vi "ADAM_scan_table.vi"() -> ()   [LabVIEW 2022 SP3]
uses:
  <vilib>/Utility/miscctls.llb/LVRowAndColumnUnsignedTypeDef.ctl
  Anemometry/Anemometry Sub Vis/Controls/Serveds.ctl
  ADAM Client/Sub VIs/ADAM Controls/Module_type_ADAM.ctl
  ADAM Client/Sub VIs/ADAM Controls/Traverse_Level_State.ctl
  Anemometry/Anemometry Sub Vis/Controls/Post_Process.ctl
  ADAM Client/Sub VIs/ADAM Controls/Channel_State.ctl
  ADAM Client/Sub VIs/ADAM Controls/Ch_description_ADAM.ctl
  ADAM Client/Sub VIs/ADAM Controls/Function_ADAM.ctl
  ADAM Client/Sub VIs/ADAM Controls/Calib_type_ADAM.ctl
  ADAM Client/Sub VIs/ADAM Controls/Address.ctl
  700e9d19-378c-4c45-b55c-3bbad4659b44.vi
  Anemometry/Anemometry Sub Vis/Globals/Preference_global.vi
  ADAM_Global.vi
  Sub VI's/Channel_Description_Global.vi
  Anemometry/Anemometry Sub Vis/Globals/Meas_global.vi
  Sub VI's/Logged_Data_real_Global.vi
  Anemometry/Anemometry Sub Vis/Globals/Gas_management_global.vi
  Anemometry/Anemometry Sub Vis/Globals/Constants_global.vi
  <vilib>/Comparison/Less/Less Functor/Less Functor.lvclass
panel:
  in  "openSetupFolder":bool
  out "Scan:Padding:(ms)":i32
  in  "launchStatus":bool
  in  "launchTiming":bool
  out "lastScan":dbl caption="Last Scan" format="%_4fs"
  out "scanNum":i32 caption="Scan Number"
  out "enunciator":string caption="Current Process"
  in  "launchEditor":bool
  in  "flushChannelErrors":bool
  in  "stopAll":bool
  out "Talking Modules":string[][](table)
  out "Channel Errors":string[][](table)
  in  "Reconfigure Gills":bool
  in  "Log full Res Data":bool
  out "Duty No":u16 format="%016b"
  in  "Save Current setup":bool=TRUE
  in  "Load setup from file":bool
  out "ADAM scan comments":string
  out "History length":i32=250
  in  "stop":bool
  out "Results":dbl[](array[numeric]) format="%.3f"
  out "Titles":string[](array[string])
  # "The default value for this\nis saved in Scan_mode.txt"
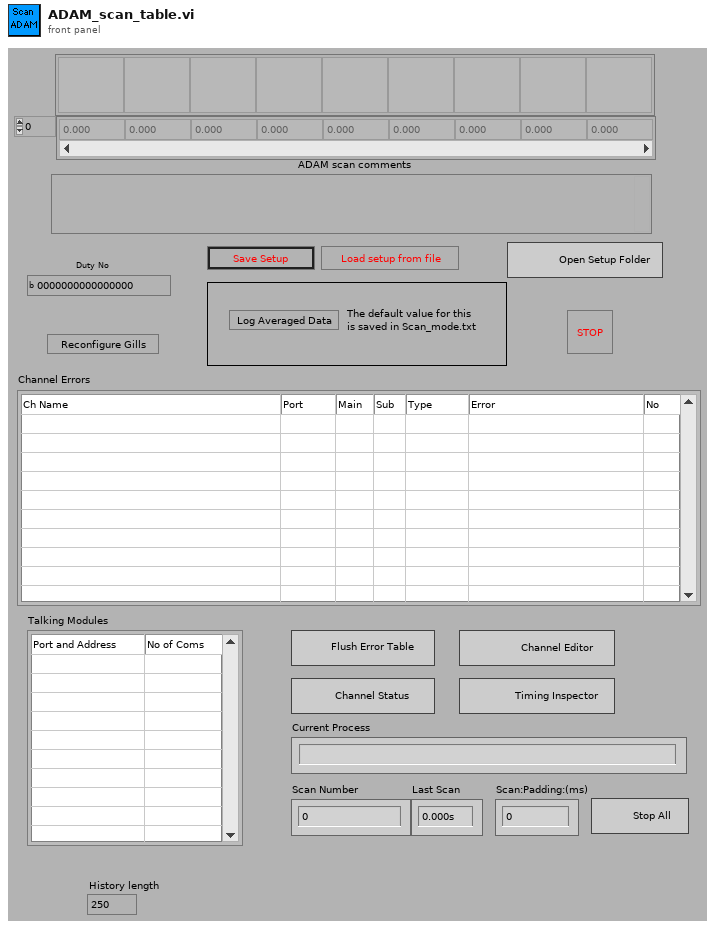
[diagram p1: front panel]
types:
  T1 = typedef "LVRowAndColumnUnsignedTypeDef.ctl" = cluster{"Row":u32, "Column":u32}
  T2 = enum16{"Load ADAM setup from excel file", "Save ADAM setup to excel file"}
  T3 = typedef "Serveds.ctl" = enum16{"Read Global", "Load Global From File"}
  T4 = typedef "Module_type_ADAM.ctl" = string
  T5 = typedef "Traverse_Level_State.ctl" = enum16{"Running", "Complete"}
  T6 = typedef "Post_Process.ctl" = enum16{"Take New Data", "Post Process Raw Data File"}
  T7 = typedef "Channel_State.ctl" = enum16{"On", "Off", "Always On", "Always Off"}
  T8 = enum32{"Invalid", "Standard", "Closed", "Hidden", "Minimized", "Maximized"}
  T9 = enum16{"Append to Global", "Read Global then Clear"}
  T10 = typedef "Ch_description_ADAM.ctl" = cluster{"Ch Name":string, "Type":T4, "Function":T11, "Ch State":T7, "Calibration type":T12, "A":dbl, "B":dbl, "C":dbl, "D":dbl, "Comments":string, "Address":T13, "String":string, "Duty":u16}
  T11 = typedef "Function_ADAM.ctl" = enum16{"Analogue Input", "Digital Input", "Event counter", "Event rate", "Analogue Output", "Digital Output", "Relay Output"}
  T12 = typedef "Calib_type_ADAM.ctl" = string
  T13 = typedef "Address.ctl" = cluster{"Main":i32, "Ch.":i32, "Sub":i32, "Port Name":string}
  T14 = enum16{"On", "Off", "Always On", "Always Off", "Delete"}
  T15 = typedef "Client_State_Cluster.ctl" = cluster{"Client Name":string, "Traverse level State":T5, "People to Email":string[], "Next Contact Time":dbl}
  T16 = typedef "LVDateTimeRec.ctl" = cluster{"fractional second":dbl, "second":i32, "minute":i32, "hour":i32, "day of month":i32, "month":i32, "year":i32, "day of week":i32, "day of year":i32, "DST":i32}
  T17 = typedef "ADAM_Comparitor.ctl" = cluster{"Ch to Monitor":string, "Channels to Kill":string, "Warn if Above":dbl, "Warn if Below":dbl, "Kill if Above":dbl, "Kill if Below":dbl, "Hysteresis Margin":dbl, "Averaging TIme (s)":dbl, "Warn Status":bool, "Kill Status":bool, "Extra Email addresses":string}
  T18 = cluster{"Channel Names":string[], "Last Updated":dbl[]}
  T19 = typedef "Update_scan_value.ctl" = cluster{"Channel Name":string, "New Value":dbl, "!Auto_Off":bool}
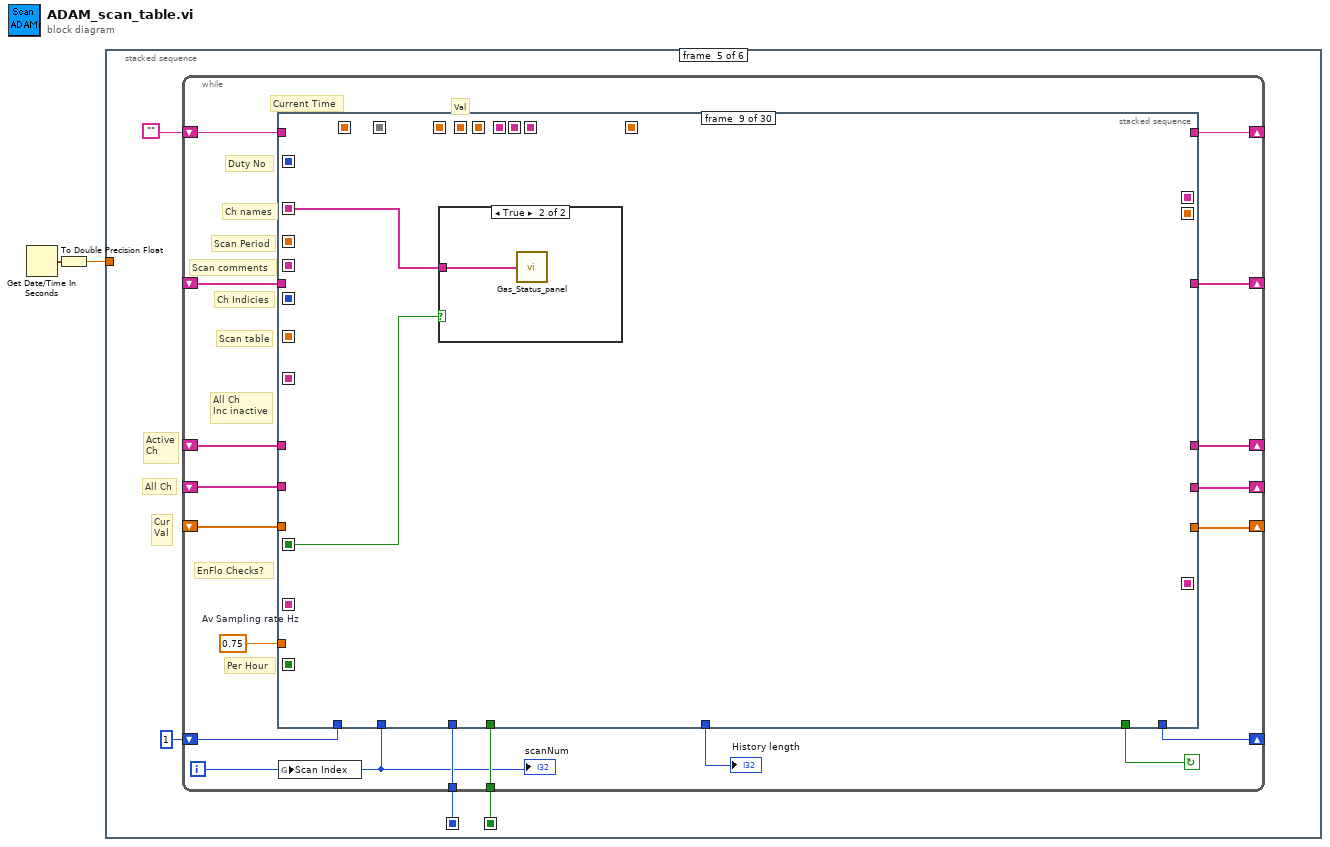
[diagram p0: block diagram]
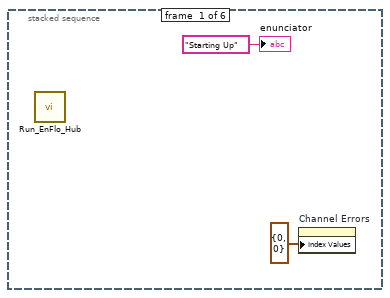
[diagram p2: hidden frame]
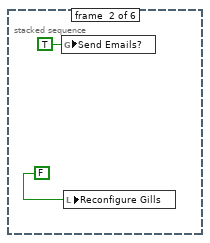
[diagram p3: hidden frame]
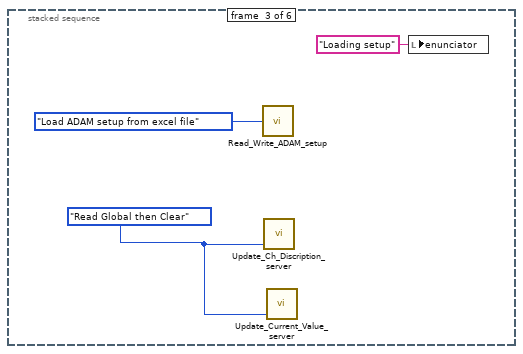
[diagram p4: hidden frame]
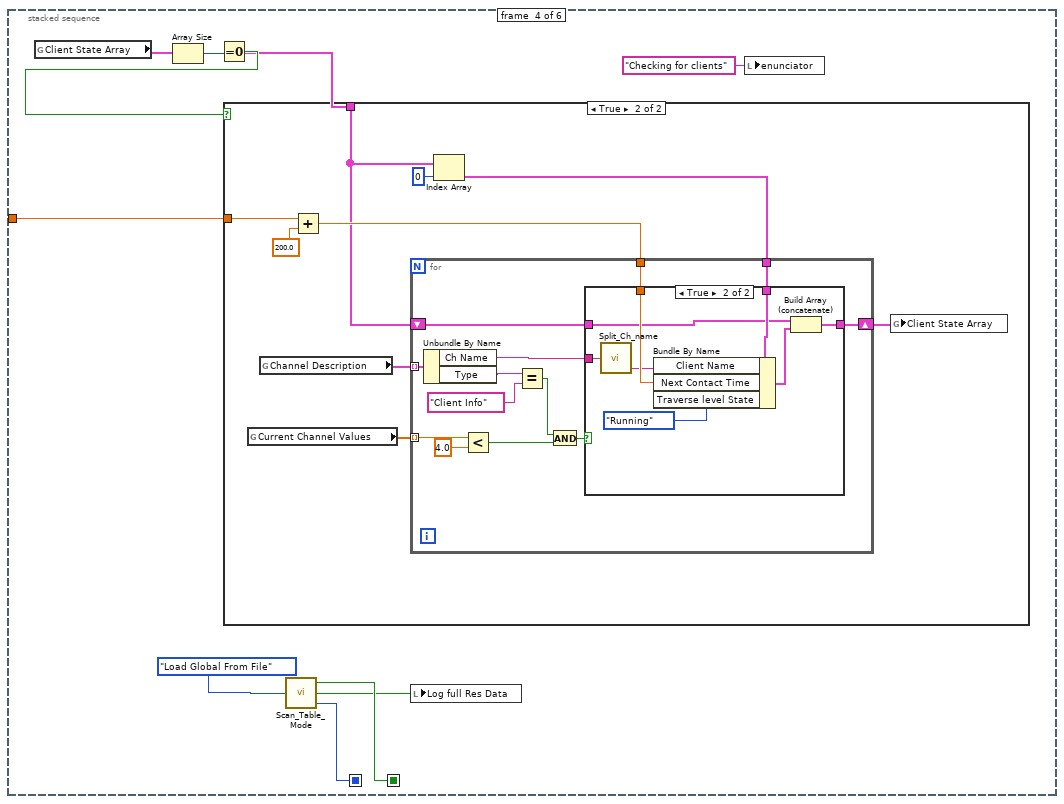
[diagram p5: hidden frame]
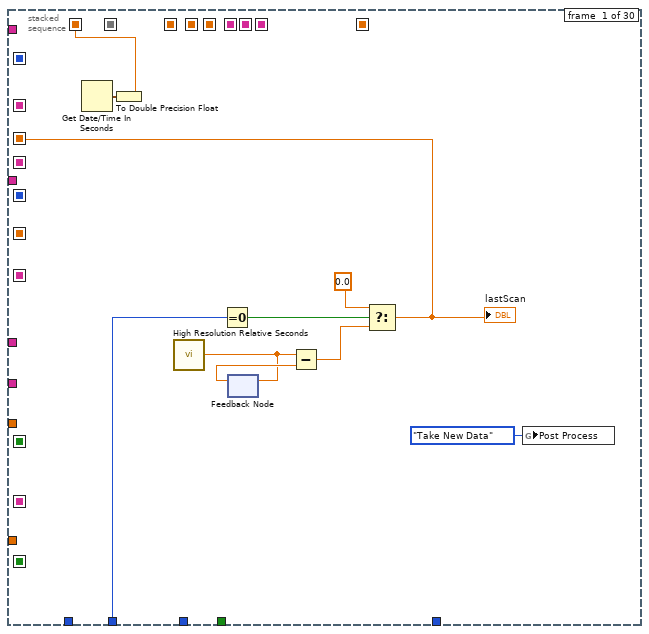
[diagram p8: hidden frame]
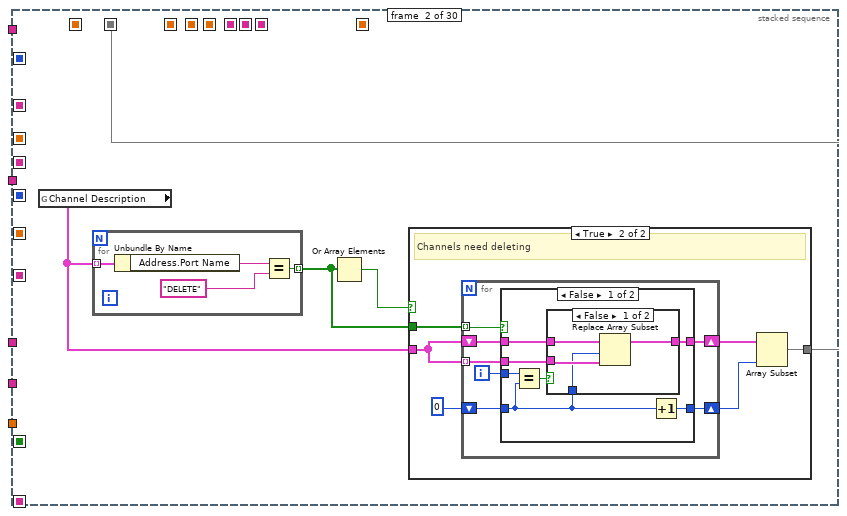
[diagram p9: hidden frame]
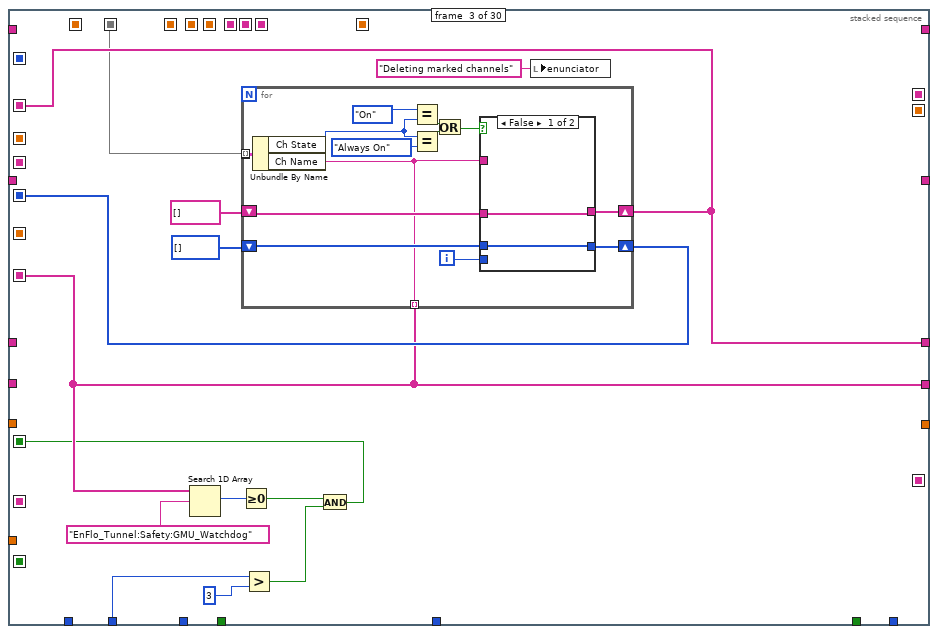
[diagram p13: hidden frame]
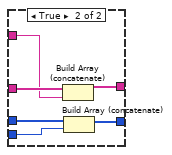
[diagram p14: hidden frame]
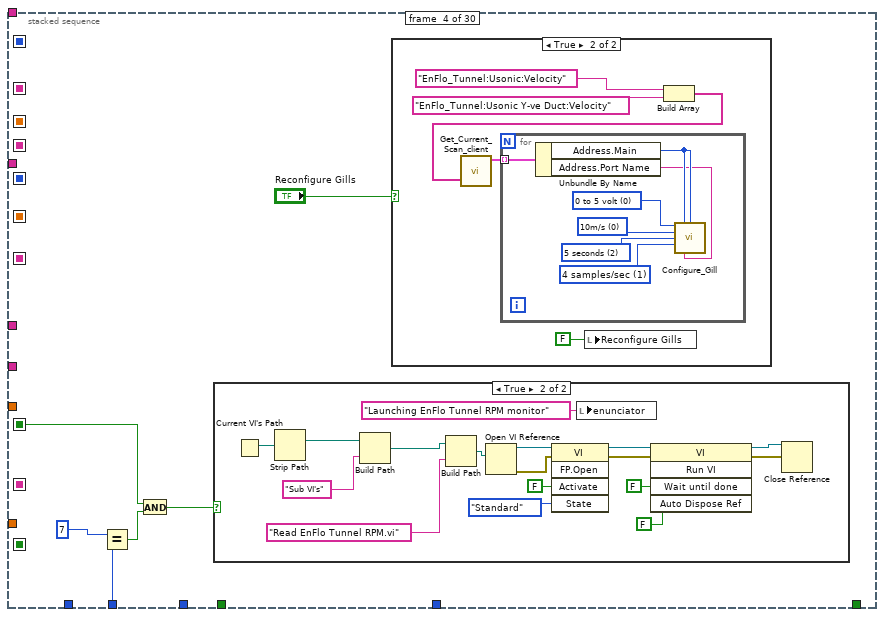
[diagram p15: hidden frame]
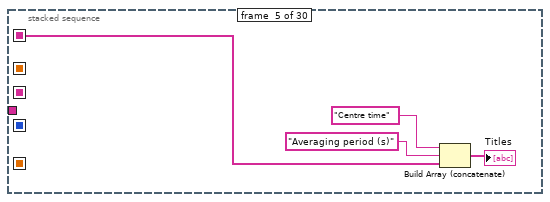
[diagram p18: hidden frame]
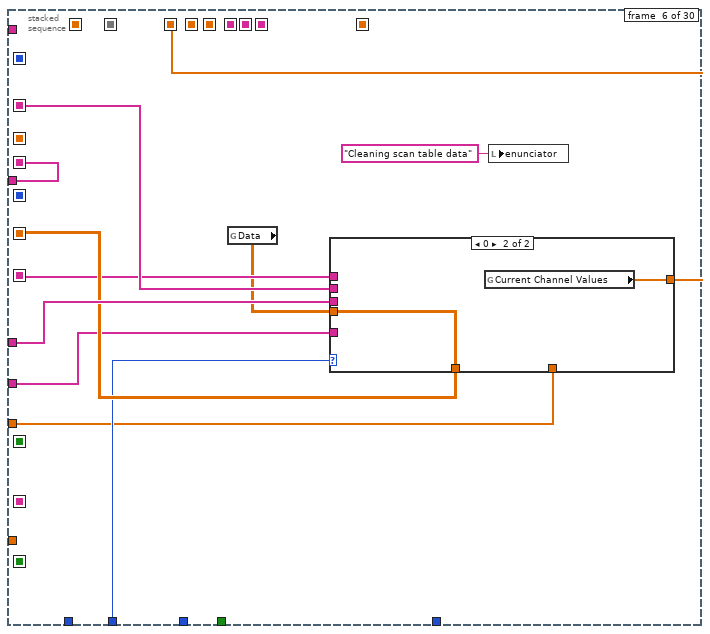
[diagram p19: hidden frame]
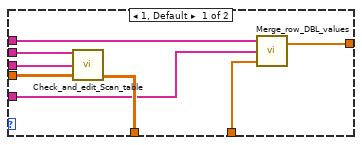
[diagram p20: hidden frame]
diagram:
  n1 = Get Date/Time In Seconds() -> (seconds since 1Jan1904=w2:timestamp)
  n2 = To Double Precision Float(number=w2) -> (double precision float=w1:dbl)
  n3 = stacked-sequence {
    seq-local: [_ _ _ w18 _ _] -> [_ _ _ _ w53 _]
    seq-local: [_ _ _ w12 _ _] -> [_ _ _ _ w51 _]
    tunnel: w1 -> [_ _ _ w11 _ _]
    frame #0 {
      n4 = call "Run_EnFlo_Hub.vi"() -> ()  [unwired: 1 in, 7 out]
      n5 = property on="Channel Errors" class="Tbl (strict)"("Index Values"=T1 {"Row"=0, "Column"=0}) -> ()  [unwired: 2 in, 2 out]
      "enunciator" <- "Starting Up" ("enunciator")
    }
    frame #1 {
      n6 = global write "Preference_global.vi" "Send Emails?"(TRUE ("Send Emails?")) -> ()
      n7 = local write "Reconfigure Gills"(FALSE ("Reconfigure Gills")) -> ()
    }
    frame #2 {
      w8 = T9."Read Global then Clear" ("Mode")
      n8 = call "Read_Write_ADAM_setup.vi"("Mode"=T2."Load ADAM setup from excel file") -> ()  [unwired: 4 out]
      n9 = call "Update_Ch_Discription_server.vi"("Mode"=w8) -> ()  [unwired: 2 in, 1 out]
      n10 = call "Update_Current_Value_server.vi"("Mode"=w8) -> ()  [unwired: 2 in, 1 out]
      n11 = local write "enunciator"("Loading setup" ("enunciator")) -> ()
    }
    frame #3 {
      n12 = global read "ADAM_Global.vi" "Client State Array"() -> (w14:T15[])
      n13 = Array Size(array=w14) -> (size(s)=w16:i32)
      n14 = Equal To 0?(x=w16) -> (x = 0?=w15:bool)
      n15 = case shown="True" w15 {
        tunnel: w14 -> [_ w20]
        tunnel: w11 -> [_ w23]
        frame False {
          # "No clients currently using server"
        }
        frame True {
          n16 = global read "ADAM_Global.vi" "Current Channel Values"() -> (w27:dbl[])
          n17 = global read "Channel_Description_Global.vi" "Channel Description"() -> (w26:T10[])
          n18 = Add(x=w23, y=200.0) -> (x+y=w21:dbl)
          n19 = Index Array(array=w20, index=0) -> (element=w24:T15)
          n20 = for {
            tunnel: w26 -> [w40] mode=indexing
            tunnel: w27 -> [w32] mode=indexing
            tunnel: w24 -> [w33]
            tunnel: w21 -> [w31]
            shift-right: [w30] -> w19
            shift-left: w20 -> [w29]
            n21 = Unbundle By Name(w40) -> ("Ch Name"=w28:string, "Type"=w37:T4)
            n22 = Less?(x=w32, y=4.0) -> (x < y?=w35:bool)
            n23 = Equal?(x=w37, y=T4 "Client Info" ("Type")) -> (x = y?=w36:bool)
            n24 = And(x=w36, y=w35) -> (x .and. y?=w34:bool)
            n25 = case shown="True" w34 {
              tunnel: w33 -> [_ w49]
              tunnel: w31 -> [_ w48]
              tunnel: [w41 w46] -> w30
              tunnel: w29 -> [w41 w45]
              tunnel: w28 -> [_ w43]
              frame False {
              }
              frame True {
                n26 = call "Split_Ch_name.vi"("Ch name"=w43) -> ("Low level"=w42:string)  [unwired: 2 out]
                n27 = Bundle By Name(cluster=w49, "Client Name"=w42, "Next Contact Time"=w48, "Traverse level State"=Traverse_Level_State."Running") -> (w44:T15)
                n28 = Build Array (concatenate)(w45, w44) -> (w46:T15[])
              }
            }
          }
          n29 = global write "ADAM_Global.vi" "Client State Array"(w19) -> ()
        }
      }
      n30 = call "Scan_Table_Mode.vi"("Mode"=Serveds."Load Global From File") -> ("Simulate Mode ?"=w18:bool, "Log Full Res Data?"=w13:bool, "Minimum Scan Period (ms)"=w12:i32)
      n31 = local write "Log full Res Data"(w13) -> ()
      n32 = local write "enunciator"("Checking for clients" ("enunciator")) -> ()
    }
    frame #4 {
      # "Active\nCh"
      # "Cur\nVal"
      # "All Ch"
      n33 = while {
        shift-left: u16 1 -> [w60]
        shift-right: [w59] -> _
        shift-left: _ -> [w61]
        shift-right: [w62] -> _
        shift-left: _ -> [w63]
        shift-right: [w64] -> _
        tunnel: w53 -> [w65]
        shift-left: _ -> [w67]
        shift-right: [w68] -> _
        shift-left: _ -> [w69]
        shift-right: [w70] -> _
        shift-right: [w57] -> _
        shift-left: "" -> [w56]
        tunnel: w51 -> [w55]
        i -> [w54]
        stop <- w71 continue-if-true
        w58 = 0.75  # Av Sampling rate Hz
        # "Per Hour"
        # "Duty No"
        # "Current Time"
        # "EnFlo Checks?"
        # "Val"
        # "All Ch\nInc inactive"
        # "Scan comments"
        # "Scan table"
        # "Ch Indicies"
        # "Ch names"
        # "Scan Period"
        n34 = stacked-sequence {
          seq-local: [_ _ _ _ _ _ _ _ _ _ _ _ _ _ _ _ _ _ w484 _ _ _ _ _ _ _ _ _ _ _] -> [_ _ _ _ _ _ _ _ _ _ _ _ _ _ _ _ _ _ _ _ w554 w586 _ _ _ _ _ w715 _ _]
          seq-local: [_ _ _ _ _ w199 _ _ _ _ _ _ _ _ _ _ _ _ _ _ _ _ _ _ _ _ _ _ _ _] -> [_ _ _ _ _ _ _ w242 _ _ _ _ _ _ _ _ _ _ _ _ _ w591 w594 _ _ _ _ _ _ _]
          seq-local: [w73 _ _ _ _ _ _ _ _ _ _ _ _ _ _ _ _ _ _ _ _ _ _ _ _ _ _ _ _ _] -> [_ _ _ _ _ _ _ _ _ _ _ _ w313 _ _ _ _ _ _ _ _ w579 _ _ _ _ _ _ _ _]
          seq-local: [_ _ _ _ _ w202 _ _ _ _ _ _ _ _ _ _ _ _ _ _ _ _ _ _ _ _ _ _ _ _] -> [_ _ _ _ _ _ _ w244 _ _ _ _ _ _ _ _ _ _ _ _ _ _ _ _ w678 _ _ _ _ _]
          seq-local: [_ _ _ _ _ _ _ _ _ _ _ _ w311 _ _ _ _ _ _ _ _ _ _ _ _ _ _ _ _ _] -> [_ _ _ _ _ _ _ _ _ _ _ _ _ _ w397 _ _ _ _ _ _ _ _ _ _ _ _ _ _ _]
          seq-local: [_ _ w130 _ _ _ _ _ _ _ _ _ _ _ _ _ _ _ _ _ _ _ _ _ _ _ _ _ _ _] -> [_ _ _ _ w190 w201 _ w245 w246 _ _ _ _ _ _ _ _ _ _ _ _ w589 _ _ _ _ _ _ _ _]
          seq-local: [_ _ w129 _ _ _ _ _ _ _ _ _ _ _ _ _ _ _ _ _ _ _ _ _ _ _ _ _ _ _] -> [_ _ _ _ _ _ w218 w240 _ w251 _ _ w312 _ _ _ _ _ _ _ _ _ w593 _ _ _ _ _ _ _]
          seq-local: [_ _ _ _ _ w195 _ _ _ _ _ _ _ _ _ _ _ _ _ _ _ _ _ _ _ _ _ _ _ _] -> [_ _ _ _ _ _ w216 w241 _ w252 w277 _ w309 _ _ _ _ _ _ _ _ _ _ _ _ _ _ _ _ _]
          seq-local: [_ _ _ _ _ _ _ _ _ _ _ _ w307 _ _ _ _ _ _ _ _ _ _ _ _ _ _ _ _ _] -> [_ _ _ _ _ _ _ _ _ _ _ _ _ _ w402 w437 _ _ w482 _ _ _ _ _ _ _ _ _ _ _]
          seq-local: [_ _ w125 _ _ _ _ _ _ _ _ _ _ _ _ _ _ _ _ _ _ _ _ _ _ _ _ _ _ _] -> [_ _ _ _ _ w197 _ w243 _ _ _ _ w308 _ w401 w436 _ _ w483 w530 w553 w588 _ _ _ _ w691 _ _ _]
          seq-local: [_ _ _ _ _ _ _ _ _ _ _ w291 _ _ _ _ _ _ _ _ _ _ _ _ _ _ _ _ _ _] -> [_ _ _ _ _ _ _ _ _ _ _ _ w306 _ w395 _ _ _ _ _ _ _ _ _ _ _ _ _ _ _]
          seq-local: [_ w82 _ _ _ _ _ _ _ _ _ _ _ _ _ _ _ _ _ _ _ _ _ _ _ _ _ _ _ _] -> [_ _ w127 _ _ _ w217 w239 _ w253 w278 _ w305 _ _ _ _ _ _ _ _ _ w592 _ _ _ _ _ _ _]
          seq-local: [w72 _ _ _ _ _ _ _ _ _ _ _ _ _ _ _ _ _ _ _ _ _ _ _ _ _ _ _ _ _] -> [_ _ _ _ _ _ _ _ _ w249 w276 _ w299 w357 w398 _ _ _ w479 _ _ w575 _ w643 _ _ _ _ _ _]
          seq-local: [_ _ _ _ _ _ _ _ _ _ _ _ _ _ _ _ _ _ _ _ _ w585 _ _ _ _ _ _ _ _] -> [_ _ _ _ _ _ _ _ _ _ _ _ _ _ _ _ _ _ _ _ _ _ w595 _ _ _ _ _ _ _]
          seq-local: [_ _ w121 _ _ _ _ _ _ _ _ _ _ _ _ _ _ _ _ _ _ _ _ _ _ _ _ _ _ _] -> [_ _ _ w154 _ _ _ _ w247 _ _ _ _ _ w400 w435 w459 _ _ _ _ _ _ _ _ _ _ _ w726 _]
          seq-local: [_ _ _ _ _ _ _ _ _ _ _ _ _ _ _ _ _ _ w481 _ _ _ _ _ _ _ _ _ _ _] -> [_ _ _ _ _ _ _ _ _ _ _ _ _ _ _ _ _ _ _ w531 _ _ _ _ _ _ _ _ _ _]
          seq-local: [_ _ _ _ _ _ w215 _ _ _ _ _ _ _ _ _ _ _ _ _ _ _ _ _ _ _ _ _ _ _] -> [_ _ _ _ _ _ _ _ _ _ _ _ w304 _ _ _ _ _ _ _ _ _ _ _ _ _ _ _ _ _]
          seq-local: [_ _ _ _ _ _ _ _ _ _ _ _ _ _ _ _ _ _ w480 _ _ _ _ _ _ _ _ _ _ _] -> [_ _ _ _ _ _ _ _ _ _ _ _ _ _ _ _ _ _ _ w529 _ _ _ _ _ _ _ _ _ _]
          seq-local: [_ _ _ _ _ _ _ _ _ _ _ _ _ _ w396 _ _ _ _ _ _ _ _ _ _ _ _ _ _ _] -> [_ _ _ _ _ _ _ _ _ _ _ _ _ _ _ w432 _ _ _ _ _ _ _ _ _ _ _ _ _ _]
          seq-local: [_ _ _ _ _ _ _ _ _ _ _ _ _ _ _ w430 _ _ _ _ _ _ _ _ _ _ _ _ _ _] -> [_ _ _ _ _ _ _ _ _ _ _ _ _ _ _ _ _ _ _ _ _ _ _ _ w666 w685 _ _ _ _]
          seq-local: [_ _ _ _ _ _ _ _ _ _ w272 _ _ _ _ _ _ _ _ _ _ _ _ _ _ _ _ _ _ _] -> [_ _ _ _ _ _ _ _ _ _ _ _ _ _ _ _ _ _ _ _ _ _ w596 w644 _ _ _ _ _ _]
          seq-local: [_ _ _ _ _ _ _ _ _ _ _ _ w303 _ _ _ _ _ _ _ _ _ _ _ _ _ _ _ _ _] -> [_ _ _ _ _ _ _ _ _ _ _ _ _ w360 _ _ _ _ _ _ _ _ _ _ _ _ _ _ _ _]
          tunnel: [_ _ _ _ _ _ _ _ _ _ _ _ _ _ _ _ _ _ _ _ _ _ _ _ _ w684 _ _ _ _] -> w71
          tunnel: [_ _ _ _ _ _ _ _ _ _ _ _ _ _ _ _ _ _ _ _ _ _ _ _ w676 _ _ _ _ _] -> w70
          tunnel: w69 -> [_ _ _ _ _ w202 _ _ _ _ _ _ _ _ _ _ _ _ _ _ _ _ _ _ _ _ _ _ _ _]
          tunnel: [_ _ w130 _ _ _ _ _ _ _ _ _ _ _ _ _ _ _ _ _ _ _ _ _ _ _ _ _ _ _] -> w68
          tunnel: w67 -> [_ _ _ _ _ w200 _ _ _ _ _ _ _ _ _ _ _ _ _ w532 _ _ _ _ _ _ _ _ _ _]
          tunnel: w54 -> [w81 _ w119 w157 _ w198 w221 _ _ _ _ _ _ _ w399 _ w455 w465 _ _ _ _ _ _ _ w689 _ _ w727 _]
          tunnel: [_ _ _ _ _ _ _ _ _ _ _ _ _ _ _ _ _ _ _ _ _ w590 _ _ _ _ _ _ _ _] -> w66
          tunnel: w65 -> [_ _ _ _ _ _ _ _ _ _ _ _ w310 _ _ _ _ _ _ _ _ _ _ _ _ _ _ _ _ _]
          tunnel: [_ _ w125 _ _ _ _ _ _ _ _ _ _ _ _ _ _ _ _ _ _ _ _ _ _ _ _ _ _ _] -> w64
          tunnel: w63 -> [_ _ _ _ _ w196 _ _ _ _ _ _ _ _ _ _ _ _ _ _ _ _ _ _ _ _ _ _ _ _]
          tunnel: [_ _ _ _ _ _ _ _ _ _ _ _ _ _ _ _ _ _ _ _ _ _ _ _ _ _ _ w715 _ _] -> w62
          tunnel: w61 -> [_ _ _ _ _ w194 _ _ _ _ _ _ _ _ _ _ _ _ _ _ _ _ _ _ _ _ _ _ _ _]
          tunnel: w60 -> [_ _ _ _ _ _ _ _ _ _ _ w292 _ _ _ _ _ _ _ _ _ _ _ _ _ _ _ _ _ _]
          tunnel: [_ _ _ _ _ _ _ _ _ _ _ w291 _ _ _ _ _ _ _ _ _ _ _ _ _ _ _ _ _ _] -> w59
          tunnel: w58 -> [_ _ _ _ _ _ w224 _ _ _ _ _ _ _ _ _ w458 w468 _ _ _ _ _ _ _ _ _ _ _ _]
          tunnel: [_ _ _ _ _ _ _ _ _ _ _ _ _ _ _ _ _ _ _ _ _ _ _ _ _ w685 _ _ _ _] -> w57
          tunnel: w56 -> [_ _ _ _ _ _ _ _ _ w250 _ _ _ _ _ _ _ _ _ _ _ _ _ _ _ _ _ _ _ _]
          tunnel: w55 -> [_ _ _ _ _ _ _ _ _ _ _ _ _ _ _ _ _ _ _ _ _ _ _ _ _ _ _ _ _ w756]
          frame #0 {
            n35 = Get Date/Time In Seconds() -> (seconds since 1Jan1904=w75:timestamp)
            n36 = To Double Precision Float(number=w75) -> (double precision float=w72:dbl)
            n37 = call <vilib>:"High Resolution Relative Seconds.vi"() -> ("relative seconds"=w77:dbl)
            n38 = Equal To 0?(x=w81) -> (x = 0?=w80:bool)
            n39 = feedback #1() -> (w78:dbl)  [unwired: 1 in]
            n40 = feedback-in #1(w77) -> ()
            n41 = Subtract(x=w77, y=w78) -> (x-y=w76:dbl)
            n42 = Select(t=0.0, s=w80, f=w76) -> (s? t:f=w73:dbl)
            "lastScan" <- w73
            n43 = global write "Meas_global.vi" "Post Process"(Post_Process."Take New Data" ("Post Process")) -> ()
          }
          frame #1 {
            n44 = global read "Channel_Description_Global.vi" "Channel Description"() -> (w84:T10[])
            n45 = for {
              tunnel: w84 -> [w117] mode=indexing
              tunnel: [w114] -> w83 mode=indexing
              n46 = Unbundle By Name(w117) -> ("Address.Port Name"=w116:string)
              n47 = Equal?(x=w116, y="DELETE") -> (x = y?=w114:bool)
            }
            n48 = Or Array Elements(Boolean array=w83) -> (logical OR=w85:bool)
            n49 = case shown="True" w85 {
              tunnel: w84 -> [w86 w90]
              tunnel: w83 -> [_ w92]
              tunnel: [w86 w87] -> w82
              frame False {
                # "Nothing to delete"
              }
              frame True {
                # "Channels need deleting"
                n50 = for {
                  shift-right: [w99] -> w89
                  shift-left: w90 -> [w98]
                  tunnel: w92 -> [w94] mode=indexing
                  shift-right: [w97] -> w88
                  shift-left: 0 -> [w95]
                  tunnel: w90 -> [w96] mode=indexing
                  i -> [w93]
                  n51 = case shown="False" w94 {
                    tunnel: [w105 w113] -> w99
                    tunnel: w98 -> [w106 w113]
                    tunnel: [w103 w112] -> w97
                    tunnel: w95 -> [w102 w112]
                    tunnel: w96 -> [w104 _]
                    tunnel: w93 -> [w101 _]
                    frame False {
                      n52 = Equal?(x=w101, y=w102) -> (x = y?=w100:bool)
                      n53 = case shown="False" w100 {
                        tunnel: w106 -> [w110 w111]
                        tunnel: [w109 w111] -> w105
                        tunnel: w104 -> [w108 _]
                        tunnel: w102 -> [w107 _]
                        frame False {
                          n54 = Replace Array Subset(array=w110, new element=w108, index=w107) -> (w109:T10[])
                        }
                        frame True {
                        }
                      }
                      n55 = Increment(x=w102) -> (x+1=w103:i32)
                    }
                    frame True {
                    }
                  }
                }
                n56 = Array Subset(array=w89, length=w88) -> (w87:T10[])  [unwired: 1 in]
              }
            }
          }
          frame #2 {
            n57 = for {
              tunnel: [w144] -> _ mode=indexing
              shift-right: [w143] -> w130
              shift-left: string[] [] -> [w134]
              shift-right: [w140] -> w129
              shift-left: i32[] [] -> [w142]
              tunnel: [w132] -> w125 mode=indexing
              tunnel: w127 -> [w144] mode=indexing
              i -> [w141]
              n58 = Unbundle By Name(w144) -> ("Ch State"=w135:T7, "Ch Name"=w132:string)
              n59 = Equal?(x=Channel_State."On" ("Channel State"), y=w135) -> (x = y?=w137:bool)
              n60 = Equal?(x=w135, y=Channel_State."Always On" ("Channel State")) -> (x = y?=w136:bool)
              n61 = Or(x=w137, y=w136) -> (x .or. y?=w133:bool)
              n62 = case shown="False" w133 {
                tunnel: w134 -> [w145 w152]
                tunnel: w132 -> [_ w151]
                tunnel: [w145 w150] -> w143
                tunnel: w142 -> [w146 w149]
                tunnel: w141 -> [_ w148]
                tunnel: [w146 w147] -> w140
                frame False {
                }
                frame True {
                  n63 = Build Array (concatenate)(w152, w151) -> (w150:string[])
                  n64 = Build Array (concatenate)(w149, w148) -> (w147:i32[])
                }
              }
            }
            n65 = Search 1D Array(1D array=w125, element="EnFlo_Tunnel:Safety:GMU_Watchdog") -> (index of element=w124:i32)  [unwired: 1 out]
            n66 = Greater Or Equal To 0?(x=w124) -> (x >= 0?=w122:bool)
            n67 = Greater?(x=w119, y=3) -> (0:w123:bool)
            n68 = And(x=w122, y=w123) -> (x .and. y?=w121:bool)
            n69 = local write "enunciator"("Deleting marked channels" ("enunciator")) -> ()
          }
          frame #3 {
            n70 = Equal?(x=7, y=w157) -> (x = y?=w155:bool)
            n71 = And(x=w154, y=w155) -> (x .and. y?=w153:bool)
            n72 = case shown="True" w153 {
              frame False {
              }
              frame True {
                n73 = Current VI's Path() -> (path=w165:path)
                n74 = Strip Path(path=w165) -> (stripped path=w162:path)  [unwired: 1 out]
                n75 = Build Path(base path=w162, name or relative path="Sub VI's") -> (appended path=w161:path)
                n76 = Build Path(base path=w161, name or relative path="Read EnFlo Tunnel RPM.vi") -> (appended path=w164:path)
                n77 = Open VI Reference(vi path=w164) -> (vi reference=w172:refnum<vi>, error out=w169:errorcluster)  [unwired: 2 in, 3 out]
                n78 = invoke class="VI" method="FP.Open"(reference=w172, error in=w169, "Activate"=FALSE ("Activate?"), "State"=T8."Standard") -> (reference out=w171:refnum<vi>, error out=w170:errorcluster)  [unwired: 1 in, 3 out]
                n79 = local write "enunciator"("Launching EnFlo Tunnel RPM monitor" ("enunciator")) -> ()
                n80 = invoke class="VI" method="Run VI"(reference=w171, error in=w170, "Wait until done"=FALSE ("Wait Until Done"), "Auto Dispose Ref"=FALSE) -> (reference out=w175:refnum<vi>, error out=w174:errorcluster)  [unwired: 1 in, 3 out]
                n81 = Close Reference(reference=w175, error in (no error)=w174) -> ()  [unwired: 1 out]
              }
            }
            n82 = case shown="True" "Reconfigure Gills" {
              frame False {
              }
              frame True {
                n83 = local write "Reconfigure Gills"(FALSE ("Reconfigure Gills")) -> ()
                n84 = Build Array("EnFlo_Tunnel:Usonic:Velocity", "EnFlo_Tunnel:Usonic Y-ve Duct:Velocity") -> (w178:string[])
                n85 = call "Get_Current_Scan_client.vi"("multipleChannels"=w178) -> ("Ch Description Array"=w177:T10[])  [unwired: 1 in, 3 out]
                n86 = for {
                  tunnel: w177 -> [w183] mode=indexing
                  w187 = u16 1 items=["1 sample/sec", "4 samples/sec"] ("Samples/sec")
                  w186 = u16 2 items=["OFF", "3 seconds", "5 seconds", "10 seconds"] ("Averaging Time")
                  w185 = u16 0 items=["10m/s", "20m/s", "30m/s", "40m/s", "50m/s", "60m/s", "70m/s"] ("Analogue O/P Scale")
                  w184 = u16 0 items=["0 to 5 volt", "+/-2.5 Volt", "4-20mA"] ("Analogue O/P Config")
                  n87 = Unbundle By Name(w183) -> ("Address.Main"=w182:i32, "Address.Port Name"=w181:string)
                  n88 = call "Configure_Gill.vi"("Analogue O/P Config"=w184, "ORIGINAL Address"=w182, "NEW Address"=w182, "Analogue O/P Scale"=w185, "Averaging Time"=w186, "Samples/sec"=w187, "Port Name"=w181) -> ()  [unwired: 9 out]
                }
              }
            }
          }
          frame #4 {
            n89 = Build Array (concatenate)("Centre time", "Averaging period (s)", w190) -> (→"Titles":string[])
          }
          frame #5 {
            n90 = global read "Logged_Data_real_Global.vi" "Data"() -> (w193:dbl[][])
            n91 = case shown="0" w198 {
              tunnel: w193 -> [w210 w212]
              tunnel: w201 -> [w207 _]
              tunnel: w200 -> [w209 _]
              tunnel: [w208 w212] -> w199
              tunnel: w197 -> [w206 _]
              tunnel: w196 -> [w205 _]
              tunnel: [w204 w211] -> w195
              tunnel: w194 -> [w203 _]
              frame 1, Default {
                n92 = call "Check_and_edit_Scan_table.vi"("2D array input"=w210, "Original Channels"=w209, "Present Channels"=w207) -> ("2D array output"=w208:dbl[][])  [unwired: 2 out]
                n93 = call "Merge_row_DBL_values.vi"("Present Row values"=w203, "Present Channels"=w205, "Desired Channels"=w206) -> ("Desired Row values"=w204:dbl[])  [unwired: 1 out]
              }
              frame 0 {
                n94 = global read "ADAM_Global.vi" "Current Channel Values"() -> (w211:dbl[])
              }
            }
            n95 = local write "enunciator"("Cleaning scan table data" ("enunciator")) -> ()
          }
          frame #6 {
            n96 = Multiply(x=w224, y=130.0) -> (x*y=w222:dbl)
            n97 = To Long Integer(number=w222) -> (32bit integer=w220:i32)
            n98 = Quotient & Remainder(x=w221, y=w220) -> (x-y*floor(x/y)=w219:i32, floor(x/y)=w214:i32)
            n99 = case shown="1, Default" w219 {
              tunnel: w218 -> [w234 _]
              tunnel: w217 -> [w233 _]
              tunnel: w216 -> [w232 _]
              tunnel: [w231 ""] -> w215
              tunnel: w214 -> [w229 _]
              tunnel: [w226 ""] -> w213
              frame 12 {
                w227 = "Re-affirming ADAM outputs" ("enunciator")
                n100 = Less?(x=w229, y=2) -> (x < y?=w230:bool)
                n101 = call "Reaffirm_ADAM_Outputs.vi"("Reset Zeros as well"=w230, "Active Ch Indicies"=w234, "Channel Description"=w233, "Current Channel Values"=w232) -> ("Scan Comments"=w235:string[])  [unwired: 2 in]
                n102 = Concatenate Strings(w235) -> (w231:string)
                n103 = local write "enunciator"(w227) -> ()
                n104 = Concatenate Strings("Done " ("string"), w227) -> (w226:string)
              }
              frame 1, Default {
              }
            }
            n105 = local write "enunciator"(w213) -> ()
          }
          frame #7 {
            n106 = global write "ADAM_Global.vi" "All Ch names"(w243) -> ()
            n107 = global write "ADAM_Global.vi" "Scan comments"(w244) -> ()
            n108 = global write "ADAM_Global.vi" "Active Ch Indicies"(w240) -> ()
            n109 = global write "Logged_Data_real_Global.vi" "Data"(w242) -> ()
            n110 = global write "ADAM_Global.vi" "Active Ch names"(w245) -> ()
            n111 = global write "Channel_Description_Global.vi" "Channel Description"(w239) -> ()
            n112 = global write "ADAM_Global.vi" "Current Channel Values"(w241) -> ()
            n113 = local write "enunciator"("Publishing to Globals" ("enunciator")) -> ()
          }
          frame #8 {
            n114 = case shown="True" w247 {
              tunnel: w246 -> [_ w248]
              frame False {
              }
              frame True {
                n115 = call "Gas_Status_panel.vi"("Ch names"=w248) -> ()  [unwired: 9 in, 6 out]
              }
            }
          }
          frame #9 {
            n116 = case shown="True" "Log full Res Data" {
              tunnel: w251 -> [_ w263]
              tunnel: w252 -> [_ w256]
              tunnel: w249 -> [_ w259]
              tunnel: w250 -> [_ w258]
              tunnel: w253 -> [_ w257]
              frame False {
              }
              frame True {
                n117 = for {
                  tunnel: w263 -> [w265] mode=indexing
                  tunnel: w257 -> [w267]
                  tunnel: [w270] -> w262 mode=indexing
                  tunnel: [w269] -> w261 mode=indexing
                  tunnel: [w268] -> w260 mode=indexing
                  tunnel: w256 -> [w266]
                  n118 = Index Array(array=w267, index=w265) -> (element=w271:T10)
                  n119 = Index Array(array=w266, index=w265) -> (element=w264:dbl)
                  n120 = Unbundle By Name(w271) -> ("Ch Name"=w268:string, "Comments"=w270:string)
                  n121 = call "Convert_No._to_String_ADAM.vi"("Input number"=w264, "Ch Description"=w271) -> ("Output sting"=w269:string)
                }
                n122 = local write "enunciator"("Logging Full-res" ("enunciator")) -> ()
                n123 = call "Write_Current_Row_to_log_file.vi"("Current Time"=w259, "Channel Names"=w260, "Channel Values"=w261, "Comments"=w262, "User added comment"=w258) -> ()  [unwired: 2 in, 1 out]
              }
            }
          }
          frame #10 {
            n124 = Seconds To Date/Time(time stamp (now)=w276) -> (date time rec=w275:T16)  [unwired: 1 in]
            n125 = Unbundle By Name(w275) -> ("hour"=w273:i32)
            n126 = feedback-in #2(w273) -> ()
            n127 = feedback #2() -> (w274:i32)  [unwired: 1 in]
            n128 = Not Equal?(x=w274, y=w273) -> (x != y?=w272:bool)
            n129 = case shown="True" w272 {
              tunnel: w277 -> [_ w280]
              tunnel: w276 -> [_ w282]
              tunnel: w278 -> [_ w281]
              frame False {
              }
              frame True {
                n130 = for {
                  tunnel: w281 -> [w287] mode=indexing
                  tunnel: [w290] -> w285 mode=indexing
                  tunnel: [w289] -> w284 mode=indexing
                  tunnel: [w288] -> w283 mode=indexing
                  tunnel: w280 -> [w286] mode=indexing
                  n131 = Unbundle By Name(w287) -> ("Ch Name"=w288:string, "Comments"=w290:string)
                  n132 = call "Convert_No._to_String_ADAM.vi"("Input number"=w286, "Ch Description"=w287) -> ("Output sting"=w289:string)
                }
                n133 = local write "enunciator"("Adding to month file" ("enunciator")) -> ()
                n134 = call "Write_All_Channels_to_Month_file.vi"("Current Time"=w282, "Channel Names"=w283, "Channel Values"=w284, "Comments"=w285) -> ()  [unwired: 3 in, 1 out]
              }
            }
          }
          frame #11 {
            # "Simplified previous code using Rotate by 1bit\nTCRL 20230324"
            n135 = Rotate(1:w292, 2:i16 1 ("y")) -> (0:w291:u16)
            "Duty No" <- w291
          }
          frame #12 {
            w296 = ";" ("element")
            # "This is where the channels actually get read"
            n136 = for {
              tunnel: w305 -> [w339]
              tunnel: w313 -> [w347]
              shift-right: [w345] -> w307
              shift-left: w309 -> [w343]
              tunnel: w308 -> [w344]
              shift-right: [w340] -> w311
              shift-left: w304 -> [w342]
              tunnel: w312 -> [w335] mode=indexing
              tunnel: w309 -> [w337]
              tunnel: w310 -> [w338]
              tunnel: w306 -> [w334]
              tunnel: [w329] -> w303 mode=indexing if=w331
              tunnel: [w328] -> w302 mode=indexing if=w327
              tunnel: w299 -> [w324]
              n137 = Index Array(array=w339, index=w335) -> (element=w333:T10)
              n138 = Index Array(array=w337, index=w335) -> (element=w336:dbl)
              n139 = Number To Decimal String(number=w324) -> (decimal integer string=w325:string)  [unwired: 1 in]
              n140 = call "Adam_Ch_Input_Output.vi"("Ch names"=w344, "Previous Scan Value"=w336, "Duty No"=w334, "Ch Description"=w333, "Scan Period"=w347, "Ch values"=w343, "Current Time (sec)"=w324, "Simulate"=w338) -> ("Calibrated units"=w346:dbl, "Good Module"=w328:string, "Error Row"=w330:string[], "Scan comment"=w341:string)  [unwired: 3 in, 1 out]
              n141 = Empty Array?(array=w330) -> (empty?=w332:bool)
              n142 = case shown="False" w332 {
                tunnel: [TRUE FALSE] -> w331
                tunnel: w330 -> [w352 w353]
                tunnel: w325 -> [w349 _]
                tunnel: [w351 w353] -> w329
                frame False {
                  n143 = Build Array (concatenate)(w352, "1", w349) -> (w351:string[])
                }
                frame True {
                }
              }
              n144 = Replace Array Subset(array=w343, new element=w346, index=w335) -> (w345:dbl[])
              n145 = Concatenate Strings(w342, w341) -> (w340:string)
              n146 = Empty String/Path?(string/path=w328) -> (empty?=w326:bool)
              n147 = Not(x=w326) -> (.not. x?=w327:bool)
            }
            n148 = call "Analyse_string_array.vi"("String array"=w302) -> ("Unique strings"=w301:string[], "Frequency"=w300:i32[])  [unwired: 1 in]
            n149 = for {
              tunnel: w301 -> [w321] mode=indexing
              tunnel: w300 -> [w323] mode=indexing
              tunnel: [w320] -> w298 mode=indexing
              tunnel: w296 -> [w319]
              n150 = Number To Decimal String(number=w323) -> (decimal integer string=w322:string)  [unwired: 1 in]
              n151 = Concatenate Strings(w321, w319, w322) -> (w320:string)
            }
            n152 = local write "enunciator"("Scanning Channels" ("initial string")) -> ()
            n153 = call "Sort 1D Array.vim"("unsorted array"=w298) -> ("sorted array"=w297:string[])  [unwired: 10 in]
            n154 = for {
              tunnel: w297 -> [w318] mode=indexing
              tunnel: w296 -> [w317]
              tunnel: [w314] -> w295 mode=indexing
              n155 = Match Pattern(string=w318, regular expression=w317) -> (before substring=w315:string, after substring=w316:string)  [unwired: 1 in, 2 out]
              n156 = Build Array(w315, w316) -> (w314:string[])
            }
            "Talking Modules" <- w295
          }
          frame #13 {
            n157 = local read "Channel Errors"() -> (w359:string[][])
            n158 = Index Array(array=w359, index (col)=0 ("disabled index (col)")) -> (element=w361:string[])  [unwired: 1 in]
            n159 = for {
              tunnel: w361 -> [w380]
              tunnel: w360 -> [w375] mode=indexing
              shift-right: [w376] -> w358
              shift-left: w359 -> [w377]
              n160 = Index Array(array=w375) -> (element=w379:string)  [unwired: 1 in]
              n161 = Search 1D Array(1D array=w380, element=w379) -> (index of element=w378:i32)  [unwired: 1 in]
              n162 = case shown="0, Default" w378 {
                selector: w378 -> [w381 _]
                tunnel: w377 -> [w391 w394]
                tunnel: [w382 w393] -> w376
                tunnel: w375 -> [w386 w392]
                frame 0, Default {
                  w385 = 6
                  n163 = Index Array(array=w391, index (row)=w381) -> (element=w388:string[])  [unwired: 1 in]
                  n164 = Index Array(array=w388, index=w385) -> (element=w387:string)
                  n165 = Decimal String To Number(string=w387) -> (number=w390:i32)  [unwired: 2 in, 1 out]
                  n166 = Increment(x=w390) -> (x+1=w389:i32)
                  n167 = Number To Decimal String(number=w389) -> (decimal integer string=w384:string)  [unwired: 1 in]
                  n168 = Replace Array Subset(array=w386, new element=w384, index=w385) -> (w383:string[])
                  n169 = Replace Array Subset(array=w391, new element=w383, index (row)=w381) -> (w382:string[][])  [unwired: 1 in]
                }
                frame -1 {
                  n170 = Build Array (concatenate)(w394, w392) -> (w393:string[][])
                }
              }
            }
            n171 = case shown="False" "flushChannelErrors" {
              tunnel: w358 -> [w365 _]
              tunnel: w357 -> [w364 _]
              tunnel: [w363 string[][] [] ("Channel Errors")] -> w356
              frame False {
                n172 = for {
                  tunnel: w365 -> [w367] mode=indexing
                  tunnel: w364 -> [w370]
                  tunnel: [w367] -> w363 mode=indexing if=w366
                  n173 = Index Array(array=w367, index=7) -> (element=w372:string)
                  n174 = Fract/Exp String To Number(string=w372) -> (number=w371:dbl)  [unwired: 3 in, 1 out]
                  n175 = Subtract(x=w370, y=w371) -> (x-y=w369:dbl)
                  n176 = Less?(x=w369, y=900.0) -> (x < y?=w366:bool)
                }
              }
              frame True {
              }
            }
            "Channel Errors" <- w356
          }
          frame #14 {
            n177 = case shown="True" w400 {
              tunnel: w402 -> [_ w409]
              tunnel: w401 -> [_ w408]
              tunnel: w399 -> [_ w406]
              tunnel: w398 -> [_ w407]
              tunnel: w397 -> [w404 w413]
              tunnel: [w404 w418] -> w396
              tunnel: w395 -> [_ w412]
              frame False {
              }
              frame True {
                n178 = global read "ADAM_Global.vi" "Comparitor Array"() -> (w417:T17[])
                n179 = for {
                  tunnel: w417 -> [w425] mode=indexing
                  tunnel: [w424] -> w416 mode=indexing
                  tunnel: w409 -> [w423]
                  tunnel: w408 -> [w422]
                  tunnel: [w421] -> w415 mode=indexing
                  n180 = call "ADAM_Comparitor.vi"("Comparator Info"=w425, "Ch names"=w422, "Present scan array"=w423) -> ("Comparator Info Out"=w424:T17, "Scan comment"=w421:string)  [unwired: 1 in]
                }
                n181 = call "Check A_Tunnel on Server.vi"("Values"=w409, "Ch Names"=w408, "Current Time"=w407, "Adam Loop Count"=w406) -> ("Scan comment"=w410:string)  [unwired: 2 in]
                n182 = call "Check D_Tunnel on Server.vi"("Values"=w409, "Ch Names"=w408, "Current Time"=w407, "Adam Loop Count"=w406) -> ("Scan comment"=w405:string)  [unwired: 2 in]
                n183 = call "LDA2_Safety.vi"("Adam Loop Count"=w406, "Ch Names"=w408, "Values"=w409) -> ("Scan comment"=w414:string)
                n184 = call "Safety_Check.vi"("Duty No"=w412, "Values"=w409, "Ch Names"=w408, "Adam Loop Count"=w406, "Current Time"=w407) -> ("Scan comment"=w420:string)
                n185 = call "Check_Aero_Tunnel_on_Server.vi"("Values"=w409, "Ch Names"=w408, "Current Time"=w407, "Adam Loop Count"=w406) -> ("Scan comment"=w419:string)  [unwired: 2 in]
                n186 = global write "ADAM_Global.vi" "Comparitor Array"(w416) -> ()
                n187 = Concatenate Strings(w413, w405, w410, w414, w420, w419, w415) -> (w418:string)
                n188 = local write "enunciator"("Doing Safety Checks" ("enunciator")) -> ()
              }
            }
            n189 = property on="Results" class="Arr (strict)"() -> ("Index Values"=w403:u32[])  [unwired: 2 in, 2 out]
            n190 = property on="Titles" class="Arr (strict)"("Index Values"=w403) -> ()  [unwired: 2 in, 2 out]
          }
          frame #15 {
            n191 = call <vilib>:"High Resolution Relative Seconds.vi"() -> ("relative seconds"=w427:dbl)
            n192 = feedback #3() -> (w426:dbl)  [unwired: 1 in]
            n193 = Subtract(x=w427, y=w426) -> (x-y=w429:dbl)
            n194 = Greater?(x=w429, y=60.0) -> (0:w433:bool)
            n195 = case shown="True" w433 {
              tunnel: w437 -> [_ w445]
              tunnel: w436 -> [_ w444]
              tunnel: w435 -> [_ w443]
              tunnel: [w439 w442] -> w431
              tunnel: w432 -> [w439 w441]
              tunnel: [w438 w440] -> w428
              tunnel: w427 -> [_ w440]
              tunnel: w426 -> [w438 _]
              frame False {
              }
              frame True {
                n196 = case shown="True" w443 {
                  tunnel: w445 -> [_ w452]
                  tunnel: w444 -> [_ w451]
                  tunnel: [w446 w449] -> w442
                  tunnel: w441 -> [w446 w450]
                  frame False {
                  }
                  frame True {
                    n197 = call "Do_Every_minute.vi"("Ch Names"=w451, "Values"=w452) -> ("Scan Comments"=w448:string)
                    n198 = local write "enunciator"("Every Minute tasks" ("enunciator")) -> ()
                    n199 = Concatenate Strings(w450, w448) -> (w449:string)
                  }
                }
              }
            }
            n200 = feedback-in #3(w428) -> ()
            n201 = call "Remove_unprintable_Char.vi"("Input String"=w431) -> ("Output String"=w430:string)
          }
          frame #16 {
            n202 = Multiply(x=w458, y=350.0) -> (x*y=w456:dbl)
            n203 = To Long Integer(number=w456) -> (32bit integer=w454:i32)
            n204 = Quotient & Remainder(x=w455, y=w454) -> (x-y*floor(x/y)=w453:i32)  [unwired: 1 out]
            n205 = case shown="0" w453 {
              tunnel: w459 -> [w460 _]
              frame 0 {
                n206 = case shown="True" w460 {
                  frame False {
                  }
                  frame True {
                    w462 = TRUE  # Set Watchdogs
                    n207 = local write "enunciator"("Kicking watchdog" ("enunciator")) -> ()
                    n208 = call "Set_Adam_Watchdogs.vi"("Set Watchdogs"=w462) -> ()  [unwired: 1 out]
                  }
                }
              }
              frame 1, Default {
              }
            }
          }
          frame #17 {
            n209 = Multiply(x=w468, y=55.0) -> (x*y=w466:dbl)
            n210 = To Long Integer(number=w466) -> (32bit integer=w464:i32)
            n211 = Quotient & Remainder(x=w465, y=w464) -> (x-y*floor(x/y)=w463:i32)  [unwired: 1 out]
            n212 = case shown="0" w463 {
              frame 0 {
                n213 = case shown="True" "Save Current setup" {
                  frame False {
                  }
                  frame True {
                    n214 = call "Read_Write_ADAM_setup.vi"("Mode"=T2."Save ADAM setup to excel file") -> ()  [unwired: 4 out]
                    n215 = local write "enunciator"("Saving setup" ("enunciator")) -> ()
                  }
                }
              }
              frame 1, Default {
              }
            }
          }
          frame #18 {
            n216 = global read "ADAM_Global.vi" "Updated Values Log"() -> (w473:T18)
            n217 = Unbundle By Name(w473) -> ("Channel Names"=w474:string[], "Last Updated"=w475:dbl[])
            n218 = call "Update_Current_Value_server.vi"("Mode"=T9."Read Global then Clear") -> ("Update array out"=w486:T19[])  [unwired: 2 in]
            n219 = for {
              tunnel: w483 -> [w501]
              tunnel: w486 -> [w496] mode=indexing
              shift-right: [w499] -> w484
              shift-left: w482 -> [w500]
              tunnel: [w492] -> w481 mode=indexing
              tunnel: [w495] -> w480 mode=indexing
              shift-right: [w491] -> w477
              shift-left: w474 -> [w493]
              shift-right: [w489] -> w478
              shift-left: w475 -> [w488]
              tunnel: w479 -> [w490]
              n220 = Unbundle By Name(w496) -> ("Channel Name"=w492:string, "New Value"=w495:dbl, "!Auto_Off"=w487:bool)
              n221 = Search 1D Array(1D array=w501, element=w492) -> (index of element=w498:i32)  [unwired: 1 out]
              n222 = Less Than 0?(x=w498) -> (x < 0?=w497:bool)
              n223 = case shown="True" w497 {
                tunnel: w492 -> [_ w517]
                tunnel: w496 -> [_ w522]
                tunnel: w487 -> [_ w516]
                frame False {
                }
                frame True {
                  n224 = call "Check_Ch_Name_colons.vi"("No of Colons"=2, "Ch Name in"=w517) -> ("Ch Name out"=w518:string)
                  n225 = global read "ADAM_Global.vi" "Update Current Value"() -> (w521:T19[])
                  n226 = Select(t="!Auto_Off", s=w516, f="") -> (s? t:f=w515:string)
                  n227 = Bundle By Name(cluster=T10 {"Ch Name"="", "Type"="Hold Value", "Function"=enum."Analogue Input", "Ch State"=enum."On", "Calibration type"="", "A"=0.0, "B"=0.0, "C"=0.0, "D"=0.0, "Comments"="", "Address"={"Main"=0, "Ch."=0, "Sub"=0, "Port Name"=""}, "String"="", "Duty"=0} ("Ch Description"), "Ch Name"=w518, "Type"=T4 "Hold Value", "Comments"=w515) -> (w526:T10)
                  n228 = Build Array (concatenate)(w521, w522) -> (w520:T19[])
                  n229 = global write "ADAM_Global.vi" "Update Current Value"(w520) -> ()
                  n230 = global read "Preference_global.vi" "Rig Setup"() -> (w524:string)
                  n231 = Build Array(w526) -> (w525:T10[])
                  n232 = call "Update_Ch_Discription_server.vi"("Mode"=T9."Append to Global", "Client HD name"=w524, "Channels to update In"=w525) -> ()  [unwired: 1 out]
                }
              }
              n233 = Replace Array Subset(array=w500, new element=w495, index=w498) -> (w499:dbl[])
              n234 = Search 1D Array(1D array=w493, element=w492) -> (index of element=w494:i32)  [unwired: 1 out]
              n235 = case shown="-1" w494 {
                selector: w494 -> [w503 _]
                tunnel: w493 -> [w506 w512]
                tunnel: w492 -> [_ w511]
                tunnel: [w506 w510] -> w491
                tunnel: w490 -> [w502 w509]
                tunnel: [w504 w508] -> w489
                tunnel: w488 -> [w505 w507]
                frame Default {
                  n236 = Replace Array Subset(array=w505, new element=w502, index=w503) -> (w504:dbl[])
                }
                frame -1 {
                  n237 = Build Array (concatenate)(w512, w511) -> (w510:string[])
                  n238 = Build Array (concatenate)(w507, w509) -> (w508:dbl[])
                }
              }
            }
            n239 = local write "enunciator"("Updating channel Descriptions and Values" ("enunciator")) -> ()
            n240 = Bundle By Name(cluster=w473, "Channel Names"=w477, "Last Updated"=w478) -> (w476:T18)
            n241 = global write "ADAM_Global.vi" "Updated Values Log"(w476) -> ()
          }
          frame #19 {
            n242 = for {
              tunnel: w532 -> [w544]
              tunnel: w531 -> [w542] mode=indexing
              tunnel: w530 -> [w543]
              tunnel: w529 -> [w538] mode=indexing
              n243 = Not Equal To 0?(x=w538) -> (x != 0?=w537:bool)
              n244 = Not A Number/Path/Refnum?(number/path/refnum=w538) -> (NaN/Path/Refnum?=w535:bool)
              n245 = Search 1D Array(1D array=w544, element=w542) -> (index of element=w541:i32)  [unwired: 1 out]
              n246 = Not(x=w535) -> (.not. x?=w534:bool)
              n247 = Or(x=w534, y=w537) -> (x .or. y?=w536:bool)
              n248 = Less Than 0?(x=w541) -> (x < 0?=w540:bool)
              n249 = And(x=w536, y=w540) -> (x .and. y?=w539:bool)
              n250 = case shown="True" w539 {
                tunnel: w543 -> [_ w552]
                tunnel: w542 -> [_ w551]
                frame False {
                }
                frame True {
                  n251 = global read "Channel_Description_Global.vi" "Channel Description"() -> (w547:T10[])
                  n252 = Search 1D Array(1D array=w552, element=w551) -> (index of element=w546:i32)  [unwired: 1 out]
                  n253 = Index Array(array=w547, index=w546) -> (element=w550:T10)
                  n254 = Bundle By Name(cluster=w550, "Ch State"=Channel_State."On") -> (w548:T10)
                  n255 = Replace Array Subset(array=w547, new element=w548, index=w546) -> (w545:T10[])
                  n256 = global write "Channel_Description_Global.vi" "Channel Description"(w545) -> ()
                }
              }
              n257 = local write "enunciator"("Turning channels On" ("enunciator")) -> ()
            }
          }
          frame #20 {
            n258 = while {
              tunnel: w554 -> [w558]
              tunnel: w553 -> [w559]
              shift-right: [w567] -> _
              shift-left: _ -> [w566]
              shift-right: [w564] -> _
              shift-left: _ -> [w565]
              stop <- TRUE stop-if-true
              n259 = Search 1D Array(1D array=w559, element="GMU1:Source:Release Temp") -> (index of element=w572:i32)  [unwired: 1 out]
              n260 = Search 1D Array(1D array=w559, element="GMU2:Source:Release Temp") -> (index of element=w557:i32)  [unwired: 1 out]
              n261 = Index Array(array=w558, index #1=w572, index #2=w557) -> (element #1=w571:dbl, element #2=w556:dbl)
              n262 = Build Array (concatenate)(w571, w566) -> (w570:dbl[])
              n263 = Build Array (concatenate)(w556, w565) -> (w561:dbl[])
              n264 = Array Subset(array=w570, length=10 ("Array Length")) -> (w567:dbl[])  [unwired: 1 in]
              n265 = Array Subset(array=w561, length=10 ("Array Length")) -> (w564:dbl[])  [unwired: 1 in]
              n266 = call "Mean_fr_NaN_data.vi"("Data"=w567) -> ("Mean value"=w568:dbl)  [unwired: 1 out]
              n267 = call "Mean_fr_NaN_data.vi"("Data"=w564) -> ("Mean value"=w563:dbl)  [unwired: 1 out]
              n268 = global write "Gas_management_global.vi" "GMU1 Release temp (deg C)"(w568) -> ()
              n269 = global write "Gas_management_global.vi" "GMU2 Release temp (deg C)"(w563) -> ()
            }
          }
          frame #21 {
            w583 = 500000  # Table size
            # "#HereItIs The magic number setting the ADAM table size"
            n270 = Get Date/Time In Seconds() -> (seconds since 1Jan1904=w581:timestamp)
            n271 = To Double Precision Float(number=w581) -> (double precision float=w578:dbl)
            n272 = Subtract(x=w578, y=w575) -> (x-y=w577:dbl)
            n273 = Divide(x=w577, y=2.0) -> (x/y=w576:dbl)
            n274 = call "Merge_row_DBL_values.vi"("Present Row values"=w586, "Present Channels"=w588, "Desired Channels"=w589) -> ("Desired Row values"=w587:dbl[])  [unwired: 1 out]
            n275 = Add(x=w575, y=w576) -> (x+y=w574:dbl)
            n276 = Build Array (concatenate)(w574, w579, w587) -> (w585:dbl[])
            "Results" <- w585
            n277 = call "Manipulate_Table.vi"("Table size"=w583, "Latest Row"=w585, "Table Input"=w591) -> ("History length"=w590:i32, "Table Output"=w584:dbl[][])  [unwired: 1 out]
            n278 = global write "Logged_Data_real_Global.vi" "Data"(w584) -> ()
            n279 = local write "enunciator"("Trimming Scan Table" ("enunciator")) -> ()
          }
          frame #22 {
            n280 = case shown="True" w596 {
              tunnel: w595 -> [_ w614]
              tunnel: w594 -> [_ w613]
              tunnel: w593 -> [_ w601]
              tunnel: w592 -> [_ w598]
              frame False {
              }
              frame True {
                w600 = 0
                # "Turn off channels which are entirely NaN over the past hour"
                n281 = Array Size(array=w613) -> (size(s)=w612:i32[])
                n282 = Index Array(array=w612) -> (element=w607:i32)  [unwired: 1 in]
                n283 = Build Array (concatenate)(w600, w600, w601) -> (w599:i32[])
                n284 = Subtract(x=w607, y=1600) -> (x-y=w610:i32)
                n285 = Greater?(x=w607, y=500) -> (0:w604:bool)
                n286 = Less Than 0?(x=w610) -> (x < 0?=w611:bool)
                n287 = Select(t=0, s=w611, f=w610) -> (s? t:f=w608:i32)
                n288 = for {
                  tunnel: w614 -> [w620] mode=indexing
                  tunnel: w613 -> [w625]
                  tunnel: w608 -> [w624]
                  tunnel: [w615] -> w603 mode=indexing if=w618
                  tunnel: w604 -> [w621]
                  tunnel: w599 -> [w617] mode=indexing
                  tunnel: w598 -> [w616]
                  i -> [w619]
                  n289 = Not A Number/Path/Refnum?(number/path/refnum=w620) -> (NaN/Path/Refnum?=w623:bool)
                  n290 = And(x=w623, y=w621) -> (x .and. y?=w622:bool)
                  n291 = case shown="True" w622 {
                    tunnel: w625 -> [_ w642]
                    tunnel: w619 -> [_ w641]
                    tunnel: w624 -> [_ w640]
                    tunnel: [FALSE w628] -> w618
                    tunnel: w617 -> [_ w636]
                    tunnel: w616 -> [_ w635]
                    tunnel: ["" w633] -> w615
                    frame False {
                    }
                    frame True {
                      n292 = Index Array(array=w642, index (col)=w641) -> (element=w639:dbl[])  [unwired: 1 in]
                      n293 = Index Array(array=w635, index=w636) -> (element=w634:T10)
                      n294 = Unbundle By Name(w634) -> ("Ch Name"=w633:string, "Ch State"=w631:T7)
                      n295 = Array Subset(array=w639, index=w640) -> (w638:dbl[])  [unwired: 1 in]
                      n296 = Not A Number/Path/Refnum?(number/path/refnum=w638) -> (NaN/Path/Refnum?=w637:bool[])
                      n297 = And Array Elements(Boolean array=w637) -> (logical AND=w632:bool)
                      n298 = Equal?(x=w631, y=Channel_State."On" ("Ch State")) -> (x = y?=w629:bool)
                      n299 = And(x=w629, y=w632) -> (x .and. y?=w628:bool)
                    }
                  }
                }
                n300 = local write "enunciator"("Turning off dead channels" ("enunciator")) -> ()
                n301 = call "Cntrl_Ch_Status_low.vi"("Mode"=T14."Off", "Channel names"=w603) -> ()  [unwired: 1 out]
              }
            }
          }
          frame #23 {
            n302 = case shown="True" w644 {
              tunnel: w643 -> [_ w656]
              frame False {
              }
              frame True {
                n303 = global read "Constants_global.vi" "ADAM setups folder"() -> (w660:path)
                n304 = Seconds To Date/Time(time stamp (now)=w656) -> (date time rec=w657:T16)  [unwired: 1 in]
                n305 = Unbundle By Name(w657) -> ("hour"=w655:i32)
                n306 = Format Into String(format string="%02d_Hr.xls", w655) -> (resulting string=w647:string)  [unwired: 2 in, 1 out]
                n307 = Build Path(base path=w660, name or relative path="Setup_Files") -> (appended path=w659:path)
                n308 = Build Path(base path=w659, name or relative path="Current Copies") -> (appended path=w649:path)
                n309 = Build Path(base path=w659, name or relative path="Selected_Filename.txt" ("Substring")) -> (appended path=w663:path)
                n310 = Read from Text File(file (use dialog)=w663) -> (text=w664:string, error out=w650:errorcluster)  [unwired: 3 in, 2 out]
                n311 = Build Path(base path=w659, name or relative path=w664) -> (appended path=w653:path)
                n312 = call <vilib>:"Create Directory Recursive.vi"("error in (no error)"=w650, "directory"=w649) -> ("error out"=w651:errorcluster, "directory copy"=w648:path)  [unwired: 3 in, 1 out]
                n313 = local write "enunciator"("Hourly backup of ADAM setup" ("enunciator")) -> ()
                n314 = Build Path(base path=w648, name or relative path=w647) -> (appended path=w646:path)
                n315 = Copy(8:w651, 9:TRUE ("overwrite (F)"), 10:w646, 11:w653) -> ()  [unwired: 1 in, 3 out]
              }
            }
          }
          frame #24 {
            w674 = 150 ("length")
            w675 = 50  # History length
            n316 = String Subset(string=w666, length (rest)=w674) -> (substring=w668:string)  [unwired: 1 out]
            n317 = String Length(string=w668) -> (length=w673:i32)
            n318 = Equal?(x=w674, y=w673) -> (x = y?=w672:bool)
            n319 = Select(t=" Clipped ", s=w672, f="") -> (s? t:f=w669:string)
            n320 = Concatenate Strings(w669, w668) -> (w667:string)
            n321 = local write "enunciator"("Cleaning comments" ("enunciator")) -> ()
            n322 = Build Array (concatenate)(w678, w667) -> (w677:string[])
            n323 = Array Size(array=w677) -> (size(s)=w680:i32)
            n324 = Subtract(x=w680, y=w675) -> (x-y=w679:i32)
            n325 = Array Subset(array=w677, index=w679) -> (w676:string[])  [unwired: 1 in]
            "ADAM scan comments" <- w666
          }
          frame #25 {
            n326 = Format Into String(format string="%s %d %s" ("Format String"), "\nScan No " ("Header message"), w689, "\r\n") -> (resulting string=w688:string)  [unwired: 2 in, 1 out]
            n327 = call "Write_out_serial_log.vi"("Header message"=w688) -> ()
            n328 = local write "enunciator"("Writing Serial Log" ("enunciator")) -> ()
            n329 = Not Or(1:"stop", 2:"stopAll") -> (0:w684:bool)
            n330 = global write "ADAM_Global.vi" "stopAll"("stopAll") -> ()
          }
          frame #26 {
            n331 = call "Update_Ch_Discription_server.vi"("Mode"=T9."Read Global then Clear") -> ("Channels to update Out"=w692:T10[])  [unwired: 2 in]
            n332 = Array Size(array=w692) -> (size(s)=w694:i32)
            n333 = Equal To 0?(x=w694) -> (x = 0?=w693:bool)
            n334 = case shown="False" w693 {
              tunnel: w691 -> [w700 _]
              tunnel: w692 -> [w699 _]
              frame False {
                n335 = global read "Channel_Description_Global.vi" "Channel Description"() -> (w698:T10[])
                n336 = for {
                  tunnel: w700 -> [w707]
                  tunnel: w699 -> [w704] mode=indexing
                  shift-right: [w703] -> w697
                  shift-left: w698 -> [w706]
                  n337 = Unbundle By Name(w704) -> ("Ch Name"=w705:string)
                  n338 = Search 1D Array(1D array=w707, element=w705) -> (index of element=w701:i32)  [unwired: 1 out]
                  n339 = Less Than 0?(x=w701) -> (x < 0?=w702:bool)
                  n340 = case shown="True" w702 {
                    tunnel: w706 -> [w711 w714]
                    tunnel: w704 -> [w710 w712]
                    tunnel: [w709 w713] -> w703
                    tunnel: w701 -> [w708 _]
                    frame False {
                      n341 = Replace Array Subset(array=w711, new element=w710, index=w708) -> (w709:T10[])
                    }
                    frame True {
                      n342 = Build Array (concatenate)(w714, w712) -> (w713:T10[])
                    }
                  }
                }
                n343 = global write "Channel_Description_Global.vi" "Channel Description"(w697) -> ()
                n344 = local write "enunciator"("Updating Channel descriptions" ("enunciator")) -> ()
              }
              frame True {
              }
            }
          }
          frame #27 {
            n345 = case shown="True" "Load setup from file" {
              frame False {
              }
              frame True {
                n346 = call "Heater_Enable_Chs.vi"("Reload from File"=TRUE) -> ()  [unwired: 3 in, 6 out]
                n347 = local write "Save Current setup"(TRUE ("Save Current setup")) -> ()
                n348 = local write "enunciator"("Reloading ADAM Setup file" ("enunciator")) -> ()
                n349 = call "Read_Write_ADAM_setup.vi"("Mode"=T2."Load ADAM setup from excel file") -> ()  [unwired: 4 out]
              }
            }
          }
          frame #28 {
            n350 = global read "Constants_global.vi" "EnFlo SW Folder"() -> (w725:path)
            n351 = case shown="2" w727 {
              tunnel: w726 -> [_ _]
              tunnel: w725 -> [w729 w736]
              tunnel: "launchEditor" -> [_ w739]
              tunnel: "launchTiming" -> [_ w738]
              tunnel: "launchStatus" -> [_ w737]
              tunnel: "openSetupFolder" -> [_ w735]
              frame 2 {
                w730 = TRUE ("runVI (F)")
                n352 = call "Load_Comparitor_Cluster.vi"() -> ()  [unwired: 12 in]
                n353 = Build Path(base path=w729, name or relative path=path "ADAM Client/ADAM client VIs/Plot_Server_Data.vi") -> (appended path=w731:path)
                n354 = Build Path(base path=w729, name or relative path=path "ADAM Server/Log_ADAM_scan_table.vi") -> (appended path=w732:path)
                n355 = local write "enunciator"("Launching Log and Plot" ("enunciator")) -> ()
                n356 = call "Open_Close_Front_Panel.ph.vi"("runVI (F)"=w730, "VI path"=w732) -> ()  [unwired: 1 in, 1 out]
                n357 = call "Open_Close_Front_Panel.ph.vi"("runVI (F)"=w730, "VI path"=w731) -> ()  [unwired: 1 in, 1 out]
              }
              frame Default {
                n358 = case shown="True" w739 {
                  tunnel: w736 -> [_ w751]
                  frame False {
                  }
                  frame True {
                    n359 = Build Path(base path=w751, name or relative path=path "ADAM Client/ADAM client VIs/EditServerChannelInteractive.vi") -> (appended path=w750:path)
                    n360 = call "Open_Close_Front_Panel.ph.vi"("runVI (F)"=TRUE, "VI path"=w750) -> ()  [unwired: 1 in, 1 out]
                  }
                }
                n361 = case shown="True" w737 {
                  tunnel: w736 -> [_ w743]
                  frame False {
                  }
                  frame True {
                    n362 = Build Path(base path=w743, name or relative path=path "ADAM Client/ADAM client VIs/Control_Channel_Status.vi") -> (appended path=w742:path)
                    n363 = call "Open_Close_Front_Panel.ph.vi"("runVI (F)"=TRUE, "VI path"=w742) -> ()  [unwired: 1 in, 1 out]
                  }
                }
                n364 = case shown="True" w738 {
                  tunnel: w736 -> [_ w747]
                  frame False {
                  }
                  frame True {
                    n365 = Build Path(base path=w747, name or relative path=path "ADAM Server/Sub VI's/scanTimingLogger.vi") -> (appended path=w746:path)
                    n366 = call "Open_Close_Front_Panel.ph.vi"("runVI (F)"=TRUE, "VI path"=w746) -> ()  [unwired: 1 in, 1 out]
                  }
                }
                n367 = case shown="True" w735 {
                  frame False {
                  }
                  frame True {
                    n368 = global read "Constants_global.vi" "ADAM setups folder"() -> (w740:path)
                    n369 = call <vilib>:"Show in File System.vi"("file or directory path"=w740) -> ()  [unwired: 10 in, 1 out]
                  }
                }
              }
            }
          }
          frame #29 {
            # "Moved to the end of the sequence to pad the scan out if required"
            # "Control the minium scan period"
            n370 = Tick Count (ms)() -> (millisecond timer value=w761:u32)
            n371 = feedback #4() -> (w760:u32)  [unwired: 1 in]
            n372 = Subtract(x=w761, y=w760) -> (x-y=w757:u32)
            n373 = To Long Integer(number=w757) -> (32bit integer=w754:i32)
            n374 = Subtract(x=w756, y=w754) -> (x-y=w758:i32)
            n375 = In Range and Coerce(upper limit=w756, x=w758, lower limit=0) -> (coerced(x)=w753:i32)  [unwired: 1 out]
            "Scan:Padding:(ms)" <- w753
            n376 = local write "enunciator"("Wait to pad scan period to minimum" ("enunciator")) -> ()
            n377 = Wait (ms)(milliseconds to wait=w753) -> (millisecond timer value=w762:u32)
            n378 = feedback-in #4(w762) -> ()
            n379 = global write "ADAM_Global.vi" "Scan:Padding:(ms)"(w753) -> ()
          }
        }
        "History length" <- w66
        n380 = global write "ADAM_Global.vi" "Scan Index"(w54) -> ()
        "scanNum" <- w54
      }
    }
    frame #5 {
      w764 = FALSE  # Set Watchdogs
      n381 = call "Set_Adam_Watchdogs.vi"("Set Watchdogs"=w764) -> ()  [unwired: 1 out]
      n382 = call "Read_Write_ADAM_setup.vi"("Mode"=T2."Save ADAM setup to excel file") -> ()  [unwired: 4 out]
      n383 = local write "enunciator"("Saving setup and stopping" ("enunciator")) -> ()
    }
  }
